vi "Marshal.vi"(8 "error in (no error)":errorcluster, 11 "int32 in":refnum<class "int64.lvclass">) -> (0 "error out":errorcluster, 2 "Buffer":u8[](array[numeric]), 3 "int32 out":refnum<class "int64.lvclass">)   [LabVIEW 2020, in "Protobuf RAW.lvlib" / "int64.lvclass"]
uses:
  int64.lvclass
  int64.lvclass/int64.ctl
  4736b2cc-328e-48c1-834c-9aec0f57f3c9.vi
  4736b2cc-328e-48c1-834c-9aec0f57f3c9.vi/0f065a35-b637-42bd-ae45-04c3465bdb97.vi
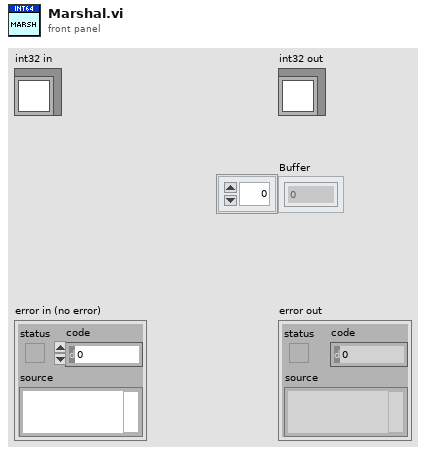
[diagram p1: front panel]
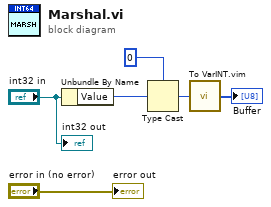
[diagram p0: block diagram]
diagram:
  n1 = Unbundle By Name("int32 in") -> ("Value"=w4:i64)
  n2 = Type Cast(type=u64 0 ("Value"), x=w4) -> (*(type *) &x=w3:u64)
  n3 = call "To VarINT.vim"("Integer"=w3) -> ("LEB128"=→"Buffer":u8[])
  "error out" <- "error in (no error)"
  "int32 out" <- "int32 in"
